vi "Conver_Coreset_Sizes_in_Percent_to_Number.vi"(6 "input cluster":T1={"Name"="", "NN"={"Name"="wrn", "No of Layers"=0, "mBatch"=1, "Layers"=[], "Dimty"=enum."In3D_Out3D", "Dims_In"={"C"=-1, "H"=-1, "W"=-1}, "Dims_Out"={"C"=-1, "H"=-1, "W"=-1}, "Working_Dir"=path "", "Train?"=FALSE, "Train_Params"={"Optimizer"=enum."SGD", "Beta_1"=0.999, "Beta_2"=0.999, "Weight Decay(L1)"=0.0, "Weight Decay(L2)"=0.0, "Data_Sampling"=enum."Random"}, "LR_Update_Policy"={"Policy_Type"=enum."Manual", "LR0"=0.0, "k"=0.0, "WarmUp_Policy"=enum."Step", "WarmUp_Iter"=100, "WarmUp_Ratio"=10.0}, "Session Data"={"Epochs"=0.0, "Tot_Iter"=1, "LR"=0.0, "LR_iter"=1}, "Ground_truth"={"Y"=variant}, "NNg_hdls"={"cudnn"=2143106709504, "cublas"=2177817002560, "stream"=2141212075440, "curand"=2143055681792}, "NN_Device"=enum."GPU", "GPU Id"=0, "Labels"=[], "Loss_Type"=enum."MSE", "Loss_Cfg_Prms"=variant, "NNG_WS"={"NNG_WS_Mem"=refnum, "Max_WS_Size"=-1}, "DryRun?"=FALSE}, "MemBank_Data"={"MemBank"=variant, "MemBank Norm"=variant}} {"NN"."LR_Update_Policy"."WarmUp_Ratio" min=1; "NN"."LR_Update_Policy"."WarmUp_Iter" min=1; "NN"."LR_Update_Policy"."LR0" format="%.7f"}, 7 "DS_Size":i32=60, 11 "Coreset_Sizes in":sgl[](array[numeric])) -> (3 "Coreset_Sizes out":i32[](array[numeric]))   [LabVIEW 2020]
uses:
  <vilib>/Ngene/DeepLTK Anomaly Detection Addon/Toolkit/API/Controls/NNPC_Instance.ctl
  <vilib>/Ngene/Deep Learning Toolkit/Toolkit/NN_Network/Controls/NN.ctl
  <vilib>/Ngene/Deep Learning Toolkit/Toolkit/NN_Layers/Controls/NN_Layer_ref.ctl
  <vilib>/Ngene/Deep Learning Toolkit/Toolkit/NN_Network/Controls/NN_In_Out_Dim-ty.ctl
  <vilib>/Ngene/Deep Learning Toolkit/Toolkit/NN_Data/API/NN_Dims(C,H,W).ctl
  <vilib>/Ngene/Deep Learning Toolkit/Toolkit/NN_Train/Controls/NN_Train_Params.ctl
  <vilib>/Ngene/Deep Learning Toolkit/Toolkit/NN_Train/Controls/NN_Train_Optimizer.ctl
  <vilib>/Ngene/Deep Learning Toolkit/Toolkit/NN_Train/Controls/NN_Train_Data_Sampling.ctl
  <vilib>/Ngene/Deep Learning Toolkit/Toolkit/NN_Train/Controls/NN_LR_Policy_Cfg.ctl
  <vilib>/Ngene/Deep Learning Toolkit/Toolkit/NN_Train/Controls/NN_LR_Policy_Type.ctl
  <vilib>/Ngene/Deep Learning Toolkit/Toolkit/NN_Train/Controls/NN_Train_Session_Data.ctl
  <vilib>/Ngene/Deep Learning Toolkit/Toolkit/NN_Data/Controls/NN_Ground_truth.ctl
  <vilib>/Ngene/Deep Learning Toolkit/Toolkit/NNg/cuda/Controls/nng_cuda_handles.ctl
  <vilib>/Ngene/Deep Learning Toolkit/Toolkit/NN_Network/Controls/NN_Device.ctl
  <vilib>/Ngene/Deep Learning Toolkit/Toolkit/NN_Train/Controls/NN_Loss_Type.ctl
  <vilib>/Ngene/Deep Learning Toolkit/Toolkit/NNg/Network/WS/Controls/NNG_WS.ctl
  <vilib>/Ngene/Deep Learning Toolkit/Toolkit/NNg/Network/WS/Controls/NNg_WS_Mem_DVR.ctl
  <vilib>/Ngene/Deep Learning Toolkit/Toolkit/NNg/cuda/Controls/cuda_Mem_desc.ctl
  <vilib>/Ngene/DeepLTK Anomaly Detection Addon/Toolkit/API/Controls/MemBank_and_Norm_Variants.ctl
  <vilib>/Ngene/Deep Learning Toolkit/Toolkit/Deep_Learning_Toolkit_by_Ngene.lvlib
  <vilib>/Ngene/DeepLTK Anomaly Detection Addon/Toolkit/DeepLTK_Anomaly_Detection_Addon.lvlib
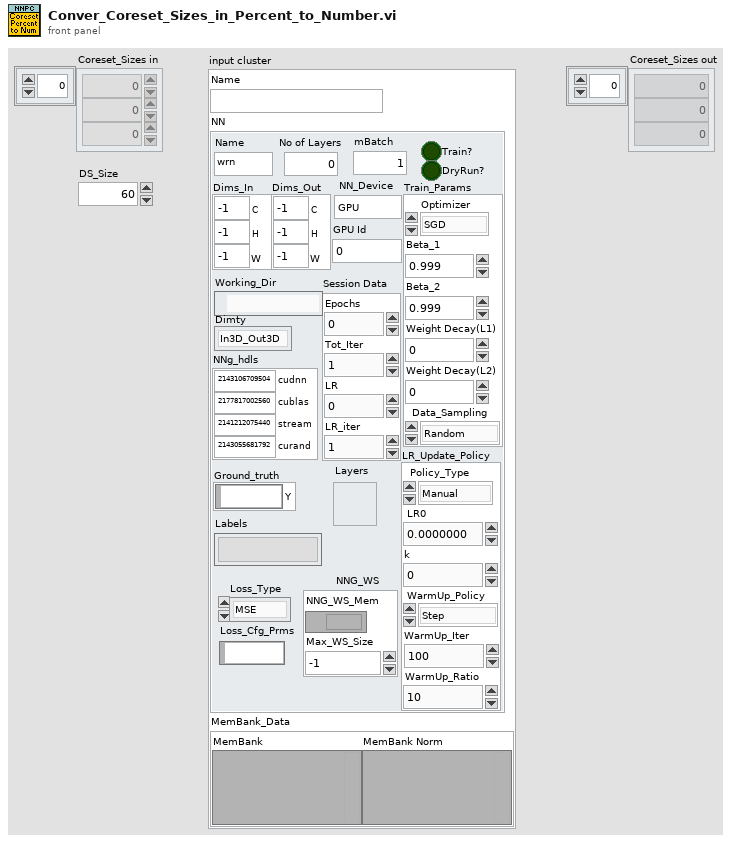
[diagram p1: front panel]
types:
  T1 = typedef "DeepLTK_Anomaly_Detection_Addon.lvlib/NNPC_Instance.ctl" = cluster{"Name":string, "NN":T2, "MemBank_Data":T18}
  T2 = typedef "Deep_Learning_Toolkit_by_Ngene.lvlib/NN.ctl" = cluster{"Name":string, "No of Layers":i32, "mBatch":i32, "Layers":T3[], "Dimty":T4, "Dims_In":T5, "Dims_Out":T5, "Working_Dir":path, "Train?":bool, "Train_Params":T6, "LR_Update_Policy":T9, "Session Data":T11, "Ground_truth":T12, "NNg_hdls":T13, "NN_Device":T14, "GPU Id":i32, "Labels":string[], "Loss_Type":T15, "Loss_Cfg_Prms":variant, "NNG_WS":T16, "DryRun?":bool}
  T3 = typedef "Deep_Learning_Toolkit_by_Ngene.lvlib/NN_Layer_ref.ctl" = refnum<file>
  T4 = typedef "Deep_Learning_Toolkit_by_Ngene.lvlib/NN_In_Out_Dim-ty.ctl" = enum8{"In1D_Out1D", "In3D_Out1D", "In3D_Out3D", "In3D_OutBBox"}
  T5 = typedef "Deep_Learning_Toolkit_by_Ngene.lvlib/NN_Dims(C,H,W).ctl" = cluster{"C":i32, "H":i32, "W":i32}
  T6 = typedef "Deep_Learning_Toolkit_by_Ngene.lvlib/NN_Train_Params.ctl" = cluster{"Optimizer":T7, "Beta_1":sgl, "Beta_2":sgl, "Weight Decay(L1)":sgl, "Weight Decay(L2)":sgl, "Data_Sampling":T8}
  T7 = typedef "Deep_Learning_Toolkit_by_Ngene.lvlib/NN_Train_Optimizer.ctl" = enum16{"SGD", "Adam", "Adagrad", "Adadelta", "RMSProp", "Nesterov"}
  T8 = typedef "Deep_Learning_Toolkit_by_Ngene.lvlib/NN_Train_Data_Sampling.ctl" = enum16{"Random", "Sequential"}
  T9 = typedef "Deep_Learning_Toolkit_by_Ngene.lvlib/NN_LR_Policy_Cfg.ctl" = cluster{"Policy_Type":T10, "LR0":dbl, "k":sgl, "WarmUp_Policy":enum16{"Step", "Ramp"}, "WarmUp_Iter":i32, "WarmUp_Ratio":sgl}
  T10 = typedef "Deep_Learning_Toolkit_by_Ngene.lvlib/NN_LR_Policy_Type.ctl" = enum16{"Manual", "Step", "Exp", "1/t"}
  T11 = typedef "Deep_Learning_Toolkit_by_Ngene.lvlib/NN_Train_Session_Data.ctl" = cluster{"Epochs":sgl, "Tot_Iter":i32, "LR":sgl, "LR_iter":i32}
  T12 = typedef "Deep_Learning_Toolkit_by_Ngene.lvlib/NN_Ground_truth.ctl" = cluster{"Y":variant}
  T13 = typedef "Deep_Learning_Toolkit_by_Ngene.lvlib/nng_cuda_handles.ctl" = cluster{"cudnn":u64, "cublas":u64, "stream":u64, "curand":u64}
  T14 = typedef "Deep_Learning_Toolkit_by_Ngene.lvlib/NN_Device.ctl" = enum16{"CPU", "GPU"}
  T15 = typedef "Deep_Learning_Toolkit_by_Ngene.lvlib/NN_Loss_Type.ctl" = enum16{"None", "MSE", "CrossEntropy", "YOLO_v2", "YOLO_v4"}
  T16 = typedef "Deep_Learning_Toolkit_by_Ngene.lvlib/NNG_WS.ctl" = cluster{"NNG_WS_Mem":T17, "Max_WS_Size":i64}
  T17 = typedef "Deep_Learning_Toolkit_by_Ngene.lvlib/NNg_WS_Mem_DVR.ctl" = refnum<data-value>
  T18 = typedef "DeepLTK_Anomaly_Detection_Addon.lvlib/MemBank_and_Norm_Variants.ctl" = cluster{"MemBank":variant, "MemBank Norm":variant}
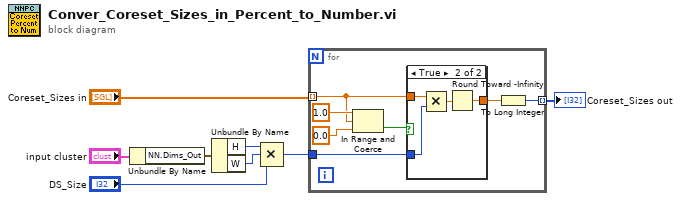
[diagram p0: block diagram]
diagram:
  n1 = Unbundle By Name("input cluster") -> ("NN.Dims_Out"=w7:T5)
  n2 = Unbundle By Name(w7) -> ("H"=w6:i32, "W"=w5:i32)
  n3 = Compound Arithmetic op=MULTIPLY(w6, w5, "DS_Size") -> (w3:i32)
  n4 = for {
    tunnel: w3 -> [w15]
    tunnel: "Coreset_Sizes in" -> [w11] mode=indexing
    tunnel: [w9] -> w2 mode=indexing
    n5 = In Range and Coerce(upper limit=sgl 1.0, x=w11, lower limit=sgl 0.0) -> (In Range?=w14:bool)  [unwired: 1 out]
    n6 = case shown="True" w14 {
      tunnel: w15 -> [_ w19]
      tunnel: w11 -> [w16 w18]
      tunnel: [w16 w17] -> w10
      frame False {
      }
      frame True {
        n7 = Multiply(x=w18, y=w19) -> (x*y=w20:sgl)
        n8 = Round Toward -Infinity(1:w20) -> (0:w17:sgl)
      }
    }
    n9 = To Long Integer(number=w10) -> (32bit integer=w9:i32)
  }
  "Coreset_Sizes out" <- w2
